vi "Status.vi"(5 "String Ref":refnum<vi>, 7 "Path":path, 10 "Error In":errorcluster, 11 "Update":string) -> (2 "Error Out":errorcluster, 3 "Output":string)   [LabVIEW 2015, in "Endigit.lvlib"]
doc: "This VI is designed to be dropped in the code wherever an error or a text update needs to be logged or displayed. No action is taken if there is no error and \"Update\" is an empty string. \n\nIf an error is input, the error's text will be formatted and added to the log specified by \"Path\" and added to a string whose reference has been input to \"String Ref\". If there is no error and \"Update\" is not an empty string, then the text of \"Update\" will be time stamped and logged to file and added to the display string. \n\n\"Path\" and \"String Ref\" can be initalized once on application start. The values will be stored on feedback nodes in the VI. Any following calls to the VI can leave these inputs unwired.\n\nThe display string will be capped at 10,000 characters.\n\nAuthored by Robert C. Mortensen\nrobert@endigit.com\n\nCopyright (c) 2015, Endigit, Inc."
uses:
  Endigit.lvlib
  <vilib>/Utility/error.llb/DialogType.ctl
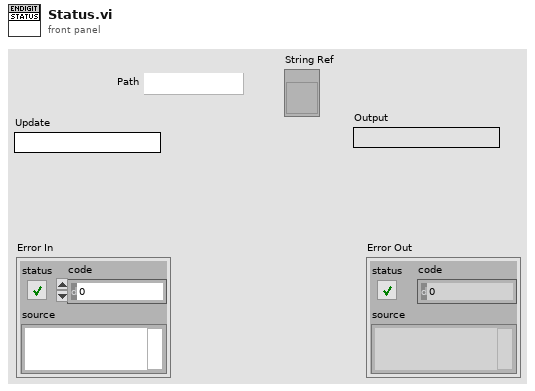
[diagram p1: front panel]
types:
  T1 = typedef "DialogType.ctl" = u16
  T2 = enum16{"open", "replace", "create", "open or create", "replace or create", "replace or create with confirmation"}
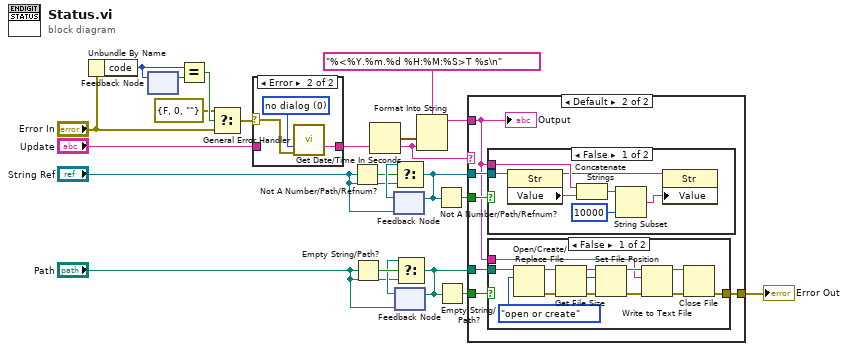
[diagram p0: block diagram]
diagram:
  n1 = Unbundle By Name("Error In") -> ("code"=w9:i32)
  n2 = feedback-in #1(w9) -> ()
  n3 = feedback #1() -> (w10:i32)  [unwired: 1 in]
  n4 = Equal?(x=w9, y=w10) -> (x = y?=w6:bool)
  n5 = Select(t=errorcluster {"status"=FALSE, "code"=0, "source"=""}, s=w6, f="Error In") -> (s? t:f=w7:errorcluster)
  n6 = case shown="Error" w7 {
    selector: w7 -> [_ w26]
    tunnel: [w23 w24] -> w11
    tunnel: "Update" -> [w23 _]
    frame No Error {
    }
    frame Error {
      w25 = T1 0 items=["no dialog", "OK message", "continue or stop message", "OK message + warnings", "continue/stop + warnings"] ("type of dialog (OK msg:1)")
      n7 = call <vilib>:"General Error Handler.vi"("type of dialog (OK msg:1)"=w25, "error in (no error)"=w26) -> ("message"=w24:string)  [unwired: 9 in, 4 out]
    }
  }
  n8 = Not A Number/Path/Refnum?(number/path/refnum="String Ref") -> (NaN/Path/Refnum?=w19:bool)
  n9 = Empty String/Path?(string/path="Path") -> (empty?=w22:bool)
  n10 = Get Date/Time In Seconds() -> (seconds since 1Jan1904=w14:timestamp)
  n11 = feedback #2("String Ref") -> (w20:refnum<vi>)
  n12 = Select(t=w20, s=w19, f="String Ref") -> (s? t:f=w15:refnum<vi>)
  n13 = feedback-in #2(w15) -> ()
  n14 = feedback #3("Path") -> (w21:path)
  n15 = Select(t=w21, s=w22, f="Path") -> (s? t:f=w17:path)
  n16 = feedback-in #3(w17) -> ()
  n17 = Format Into String(format string="%<%Y.%m.%d %H:%M:%S>T %s\n" ("x"), w14, w11) -> (resulting string=w13:string)  [unwired: 2 in, 1 out]
  n18 = Not A Number/Path/Refnum?(number/path/refnum=w15) -> (NaN/Path/Refnum?=w16:bool)
  n19 = Empty String/Path?(string/path=w17) -> (empty?=w18:bool)
  n20 = case shown="Default" w11 {
    tunnel: w18 -> [_ w32]
    tunnel: w17 -> [_ w31]
    tunnel: w16 -> [_ w30]
    tunnel: w15 -> [_ w29]
    tunnel: w13 -> [_ w28]
    tunnel: [_ w27] -> w4
    frame "" {
    }
    frame Default {
      n21 = case shown="False" w30 {
        tunnel: w29 -> [w39 _]
        tunnel: w28 -> [w37 _]
        frame False {
          n22 = property class="Str"(reference=w39) -> (reference out=w35:refnum<vi>, "Value"=w38:string)  [unwired: 1 in, 1 out]
          n23 = Concatenate Strings(w37, w38) -> (w36:string)
          n24 = String Subset(string=w36, length (rest)=10000 ("x")) -> (substring=w34:string)  [unwired: 1 in]
          n25 = property class="Str"(reference=w35, "Value"=w34) -> ()  [unwired: 1 in, 2 out]
        }
        frame True {
        }
      }
      n26 = case shown="False" w32 {
        tunnel: w31 -> [w42 _]
        tunnel: w28 -> [w40 _]
        tunnel: [w41 _] -> w27
        frame False {
          n27 = Open/Create/Replace File(file path (use dialog)=w42, operation (0:open)=T2."open or create") -> (refnum out=w51:refnum<file>, error out=w50:errorcluster)  [unwired: 4 in, 1 out]
          n28 = Get File Size(file=w51, error in=w50) -> (refnum out=w49:refnum<file>, size (in bytes)=w43:i64, 0:w48:errorcluster)
          n29 = Set File Position(offset (in bytes) (0)=w43, refnum=w49, error in=w48) -> (refnum out=w46:refnum<file>, error out=w47:errorcluster)  [unwired: 1 out]
          n30 = Write to Text File(file (use dialog)=w46, text=w40, error in=w47) -> (refnum out=w44:refnum<file>, error out=w45:errorcluster)  [unwired: 2 out]
          n31 = Close File(refnum=w44, error in=w45) -> (error out=w41:errorcluster)  [unwired: 1 out]
        }
        frame True {
        }
      }
      "Output" <- w28
    }
  }
  "Error Out" <- w4
